vi "_Remote Get Leybold Info.vi"(2 "#Index(18)":u8=18, 3 "TemplateTelegram":string="\u0002\u0016\u0000a9\u0000\u0000\u0000\u0000\u0000\u0000\u0004\u0001\u0000\u0000\u0000\u0000\u0000\u0000\u0000\u0000\u0000\u0000I") -> (1 "Reply":string="M")   [LabVIEW 2012]
panel:
  out "Array":string[](array[string])
  out "Telegram (24 bytes in Hex)":u8[](array[numeric])=[2, 22, 0, 97, 57, 0, 0, 0, 0, 0, 0, 4, 1, 0, 0, 0, 0, 0, 0, 0, 0, 0, 0, 73] format="%02x"
  # "byte-0"
  # "byte-23"
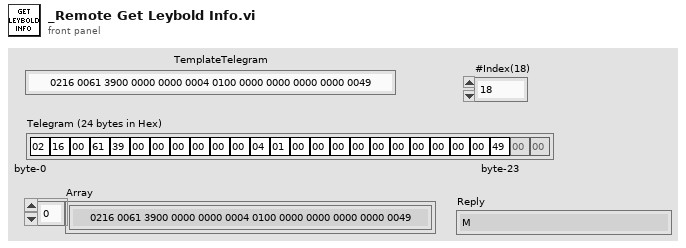
[diagram p1: front panel]
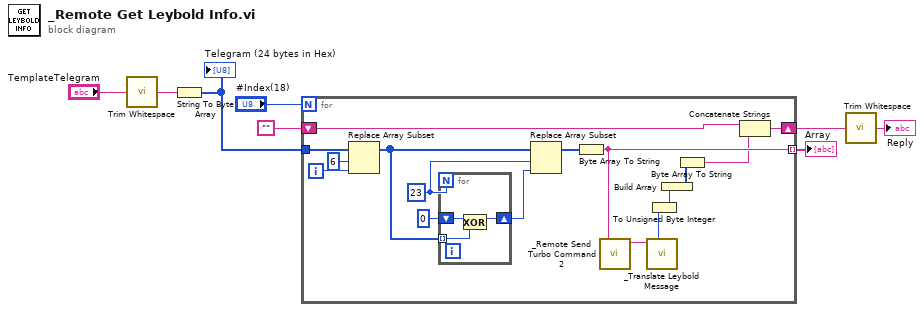
[diagram p0: block diagram]
diagram:
  n1 = call <vilib>:"Trim Whitespace.vi"("string"="TemplateTelegram") -> ("trimmed string"=w7:string)  [unwired: 1 in]
  n2 = String To Byte Array(string=w7) -> (unsigned byte array=w5:u8[])
  "Telegram (24 bytes in Hex)" <- w5
  n3 = for {
    N: "#Index(18)" -> [_]
    tunnel: w5 -> [w23]
    tunnel: [w16] -> w4 mode=indexing
    shift-right: [w11] -> w2
    shift-left: "" -> [w10]
    i -> [w22]
    w20 = 23
    n4 = Replace Array Subset(array=w23, new element=w22, index=6) -> (w18:u8[])
    n5 = for {
      N: w20 -> [_]
      tunnel: w18 -> [w26] mode=indexing
      shift-right: [w25] -> w19
      shift-left: u8 0 -> [w27]
      n6 = Exclusive Or(1:w26, 2:w27) -> (0:w25:u8)
    }
    n7 = Replace Array Subset(array=w18, new element=w19, index=w20) -> (w17:u8[])
    n8 = Byte Array To String(unsigned byte array=w17) -> (string=w16:string)
    n9 = call "_Remote Send Turbo Command 2.vi"("Telegram"=w16) -> ("Raw Reply"=w15:string)  [unwired: 5 in, 1 out]
    n10 = call "_Translate Leybold Message.vi"("LeyboldMessage"=w15) -> ("Parameter"=w14:u32)  [unwired: 3 in, 7 out]
    n11 = To Unsigned Byte Integer(number=w14) -> (unsigned 8bit integer=w12:u8)
    n12 = Build Array(w12) -> (w13:u8[])
    n13 = Byte Array To String(unsigned byte array=w13) -> (string=w9:string)
    n14 = Concatenate Strings(w10, w9) -> (w11:string)
  }
  "Array" <- w4
  n15 = call <vilib>:"Trim Whitespace.vi"("string"=w2) -> ("trimmed string"=→"Reply":string)  [unwired: 1 in]
